vi "Wave-Write Chunk Info.vi"(8 "error in (no error)":errorcluster, 9 "Size":u32=1, 10 "ID":string, 11 "refnum":refnum<file>) -> (0 "error out":errorcluster, 3 "refnum out":refnum<file>)   [LabVIEW 2020]
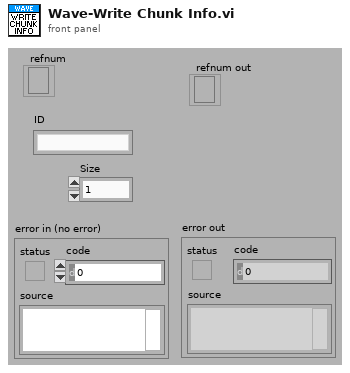
[diagram p1: front panel]
types:
  T1 = enum16{"big-endian, network order", "native, host order", "little-endian"}
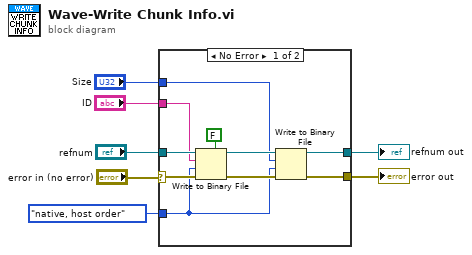
[diagram p0: block diagram]
diagram:
  n1 = case shown="No Error" "error in (no error)" {
    selector: "error in (no error)" -> [w16 w18]
    tunnel: "refnum" -> [w17 w19]
    tunnel: [w11 w19] -> w6
    tunnel: [w10 w18] -> w2
    tunnel: "ID" -> [w14 _]
    tunnel: T1."native, host order" ("byte order (0:big-endian, network order)") -> [w8 _]
    tunnel: "Size" -> [w9 _]
    frame No Error {
      n2 = Write to Binary File(file (use dialog)=w17, data=w14, error in=w16, 5:FALSE ("prepend array or string size? (T)"), 9:w8) -> (refnum out=w12:refnum<file>, error out=w13:errorcluster)  [unwired: 1 in, 1 out]
      n3 = Write to Binary File(file (use dialog)=w12, data=w9, error in=w13, 9:w8) -> (refnum out=w11:refnum<file>, error out=w10:errorcluster)  [unwired: 2 in, 1 out]
    }
    frame Error {
    }
  }
  "error out" <- w2
  "refnum out" <- w6
